vi "Find Mutual Viewing angle from GB DoF.vi"(10 "Viewing Angle Tolerance (Deg)":dbl=5.0, 11 "Grain Boundary Macro DoF":T1={"Grain 1 Orientation"=[1.0, 0.8858401549498205, 0.0], "Grain 2 Orientation"=[1.0, 0.3745791306245927, 0.0], "Twist Angle (Deg)"=0.0}) -> (1 "STEM Viewable?":bool, 2 "STEM Viewing Angles":dbl[][](array[numeric]), 3 "Mutual Viewing Angle":dbl[](array[numeric])=[1.0, -1.0, 0.0])   [LabVIEW 2010]
uses:
  <vilib>/Analysis/baseanly.llb/A x Vector.vi
  <vilib>/Analysis/NI_AALBase.lvlib
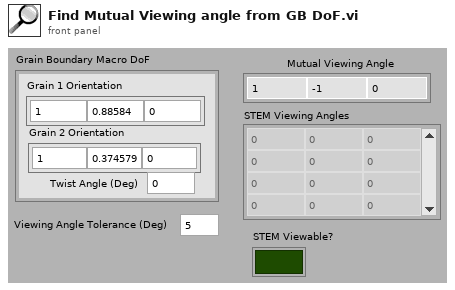
[diagram p1: front panel]
types:
  T1 = cluster{"Grain 1 Orientation":dbl[], "Grain 2 Orientation":dbl[], "Twist Angle (Deg)":dbl}
  T2 = typedef "NI_Matrix.lvlib/RealMatrix.ctl" = dbl[][]
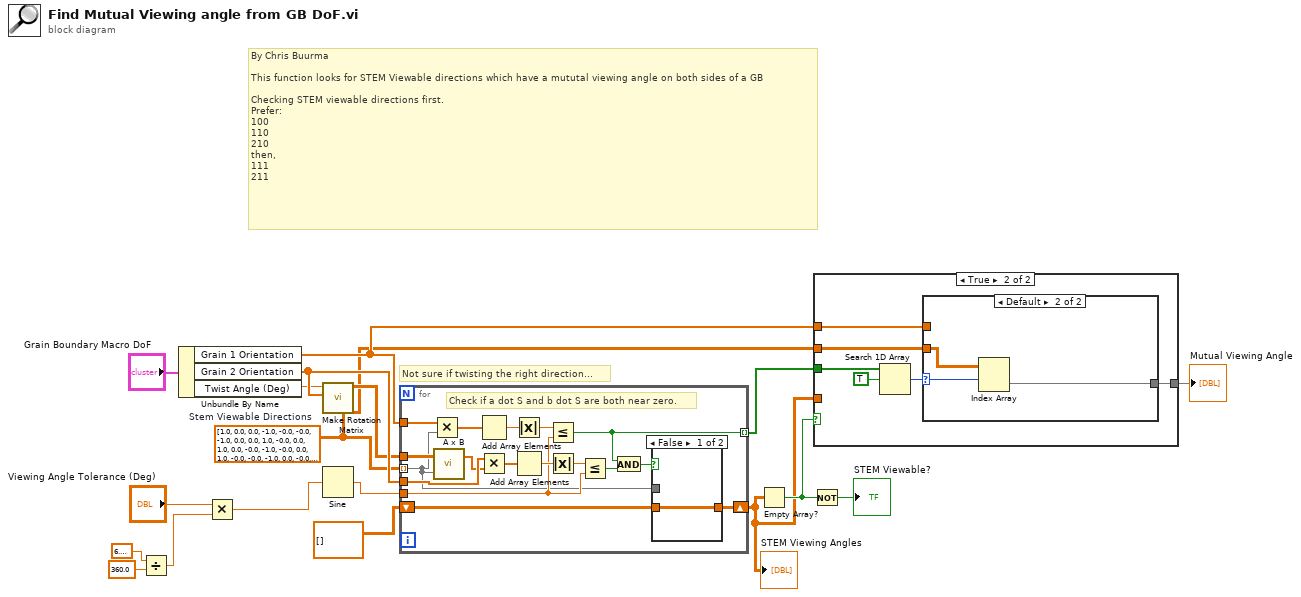
[diagram p0: block diagram]
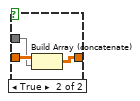
[diagram p2: hidden frame]
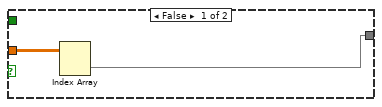
[diagram p3: hidden frame]
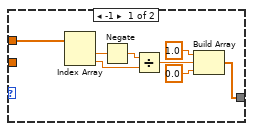
[diagram p4: hidden frame]
diagram:
  w1 = dbl[][] [[1.0, 0.0, 0.0], [-1.0, -0.0, -0.0], [-1.0, 0.0, 0.0], [1.0, -0.0, 0.0], [1.0, 0.0, -0.0], [-1.0, -0.0, 0.0], [1.0, -0.0, -0.0], [-1.0, 0.0, -0.0], [0.0, 1.0, 0.0], [-0.0, -1.0, -0.0], [-0.0, 1.0, 0.0], [0.0, -1.0, 0.0], [0.0, 1.0, -0.0], [-0.0, -1.0, 0.0], [0.0, -1.0, -0.0], [-0.0, 1.0, -0.0], [0.0, 0.0, 1.0], [-0.0, -0.0, -1.0], [-0.0, 0.0, 1.0], [0.0, -0.0, 1.0], [0.0, 0.0, -1.0], [-0.0, -0.0, 1.0], [0.0, -0.0, -1.0], [-0.0, 0.0, -1.0], [1.0, 1.0, 0.0], [-1.0, -1.0, -0.0], [-1.0, 1.0, 0.0], [1.0, -1.0, 0.0], [1.0, 1.0, -0.0], [-1.0, -1.0, 0.0], [1.0, -1.0, -0.0], [-1.0, 1.0, -0.0], [0.0, 1.0, 1.0], [-0.0, -1.0, -1.0], [-0.0, 1.0, 1.0], [0.0, -1.0, 1.0], [0.0, 1.0, -1.0], [-0.0, -1.0, 1.0], [0.0, -1.0, -1.0], [-0.0, 1.0, -1.0], [1.0, 0.0, 1.0], [-1.0, -0.0, -1.0], [-1.0, 0.0, 1.0], [1.0, -0.0, 1.0], [1.0, 0.0, -1.0], [-1.0, -0.0, 1.0], [1.0, -0.0, -1.0], [-1.0, 0.0, -1.0], [2.0, 1.0, 0.0], [-2.0, -1.0, -0.0], [-2.0, 1.0, 0.0], [2.0, -1.0, 0.0], [2.0, 1.0, -0.0], [-2.0, -1.0, 0.0], [2.0, -1.0, -0.0], [-2.0, 1.0, -0.0], [0.0, 2.0, 1.0], [-0.0, -2.0, -1.0], [-0.0, 2.0, 1.0], [0.0, -2.0, 1.0], [0.0, 2.0, -1.0], [-0.0, -2.0, 1.0], [0.0, -2.0, -1.0], [-0.0, 2.0, -1.0], [1.0, 0.0, 2.0], [-1.0, -0.0, -2.0], [-1.0, 0.0, 2.0], [1.0, -0.0, 2.0], [1.0, 0.0, -2.0], [-1.0, -0.0, 2.0], [1.0, -0.0, -2.0], [-1.0, 0.0, -2.0]]  # Stem Viewable Directions
  # "Not sure if twisting the right direction..."
  # "By Chris Buurma\n\nThis function looks for STEM Viewable directions which have a mututal viewing angle on both sides of a GB\n\nChecking STEM viewable directions first.\nPrefer: \n100\n110\n210\nthen,\n111\n211"
  n1 = Divide(x=6.283185307179586, y=360.0) -> (x/y=w6:dbl)
  n2 = Unbundle By Name("Grain Boundary Macro DoF") -> ("Grain 1 Orientation"=w15:dbl[], "Grain 2 Orientation"=w16:dbl[], "Twist Angle (Deg)"=w13:dbl)
  n3 = Multiply(x="Viewing Angle Tolerance (Deg)", y=w6) -> (x*y=w5:dbl)
  n4 = call "Make Rotation Matrix.vi"("Rotation Axis"=w16, "Rotation Angle (Degree)"=w13) -> ("Rotation Matrix"=w3:T2)  [unwired: 9 in]
  n5 = Sine(x=w5) -> (sin(x)=w4:dbl)
  n6 = for {
    tunnel: w15 -> [w35]
    tunnel: w1 -> [w20] mode=indexing
    tunnel: w16 -> [w32]
    tunnel: [w27] -> w12 mode=indexing
    tunnel: w4 -> [w25]
    shift-right: [w23] -> w2
    shift-left: dbl[][] [] -> [w22]
    tunnel: w3 -> [w21]
    # "Check if a dot S and b dot S are both near zero."
    n7 = Multiply(x=w35, y=w20) -> (x*y=w34:dbl[])
    n8 = call-poly <vilib>:"A x B.vi"("Vector"=w20, "A"=w21) -> ("A x Vector"=w19:dbl[])  [unwired: 1 out]
    n9 = Add Array Elements(numeric array=w34) -> (sum=w31:dbl)
    n10 = Multiply(x=w32, y=w19) -> (x*y=w33:dbl[])
    n11 = Absolute Value(x=w31) -> (abs(x)=w29:dbl)
    n12 = Add Array Elements(numeric array=w33) -> (sum=w30:dbl)
    n13 = Less Or Equal?(x=w29, y=w25) -> (x <= y?=w27:bool)
    n14 = Absolute Value(x=w30) -> (abs(x)=w28:dbl)
    n15 = Less Or Equal?(x=w28, y=w25) -> (x <= y?=w26:bool)
    n16 = And(x=w27, y=w26) -> (x .and. y?=w24:bool)
    n17 = case shown="False" w24 {
      tunnel: [w36 w37] -> w23
      tunnel: w22 -> [w36 w39]
      tunnel: w20 -> [_ w38]
      frame False {
      }
      frame True {
        n18 = Build Array (concatenate)(w39, w38) -> (w37:dbl[][])
      }
    }
  }
  "STEM Viewing Angles" <- w2
  n19 = Empty Array?(array=w2) -> (empty?=w10:bool)
  n20 = Not(x=w10) -> (.not. x?=→"STEM Viewable?":bool)
  n21 = case shown="True" w10 {
    tunnel: [w40 w45] -> w18
    tunnel: w12 -> [_ w47]
    tunnel: w2 -> [w41 _]
    tunnel: w15 -> [_ w43]
    tunnel: w1 -> [_ w42]
    frame False {
      n22 = Index Array(array=w41) -> (element=w40:dbl[])  [unwired: 2 in]
    }
    frame True {
      n23 = Search 1D Array(1D array=w47, element=TRUE) -> (index of element=w44:i32)  [unwired: 1 in]
      n24 = case shown="Default" w44 {
        selector: w44 -> [_ w57]
        tunnel: [w48 w58] -> w45
        tunnel: w43 -> [w53 _]
        tunnel: w42 -> [_ w56]
        frame -1 {
          n25 = Index Array(array=w53) -> (element #1=w52:dbl, element #2=w50:dbl)  [unwired: 2 in]
          n26 = Negate(x=w52) -> (-x=w51:dbl)
          n27 = Divide(x=w51, y=w50) -> (x/y=w49:dbl)
          n28 = Build Array(1.0 ("element"), w49, 0.0 ("element")) -> (w48:dbl[])
        }
        frame Default {
          n29 = Index Array(array=w56, index (row)=w57) -> (element=w58:dbl[])  [unwired: 1 in]
        }
      }
    }
  }
  "Mutual Viewing Angle" <- w18
